vi "DeltaRamp_globals.vi"() -> ()   [LabVIEW 2013]
panel:
  out "Remote_Save_String":string
  out "Remote_Save_Directory":path
  out "Remote_Req_Stop":bool
  out "Remote_Measure":bool
  out "Remote_Reset":bool
  out "Remote_Ramp_Path":path
  out "Remote_Ramp_Save":bool
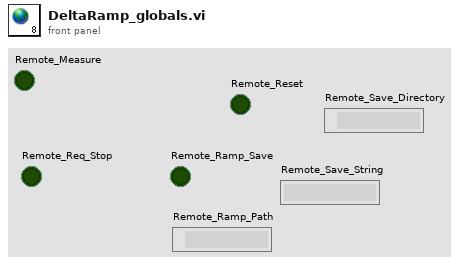
[diagram p1: front panel]
diagram:
